vi "wait_.vi"(7 "milliseconds to wait":u32, 10 "error in":errorcluster) -> (2 "error out":errorcluster)   [LabVIEW 2023, in "QR 10X Eastwood.lvlib"]
uses:
  <instrlib>/QR 10X Eastwood/QR 10X Eastwood.lvlib
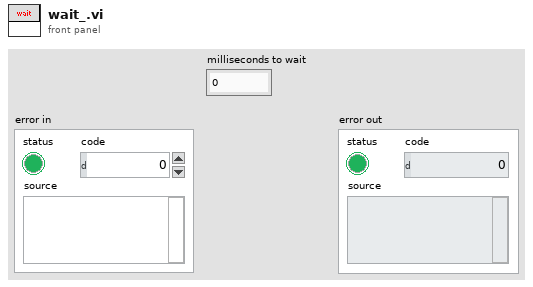
[diagram p1: front panel]
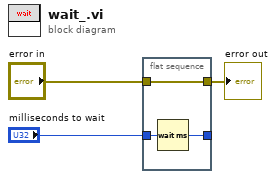
[diagram p0: block diagram]
diagram:
  n1 = flat-sequence {
    tunnel: "milliseconds to wait" -> [w6]
    tunnel: [w5] -> _
    tunnel: [w4] -> w1
    tunnel: "error in" -> [w4]
    frame #0 {
      n2 = Wait (ms)(milliseconds to wait=w6) -> (millisecond timer value=w5:u32)
    }
  }
  "error out" <- w1
